vi "Version Utility - Top level.vi"() -> ()   [LabVIEW 2014]
uses:
  <vilib>/Utility/miscctls.llb/LVRowAndColumnTypeDef.ctl
  <vilib>/Utility/cursorutil.llb/Set Cursor (Icon Pict).vi
panel:
  in  "Open Button":bool
  in  "VI Paths and version information":i32(listbox)
  in  "Stop Button":bool
  out "Parent Path":path caption="selected path"
  out "Files Processed":i32
  out "file paths":path[](array[path])
  out "VI Versions":string[][](array[string])
  out "error out":errorcluster
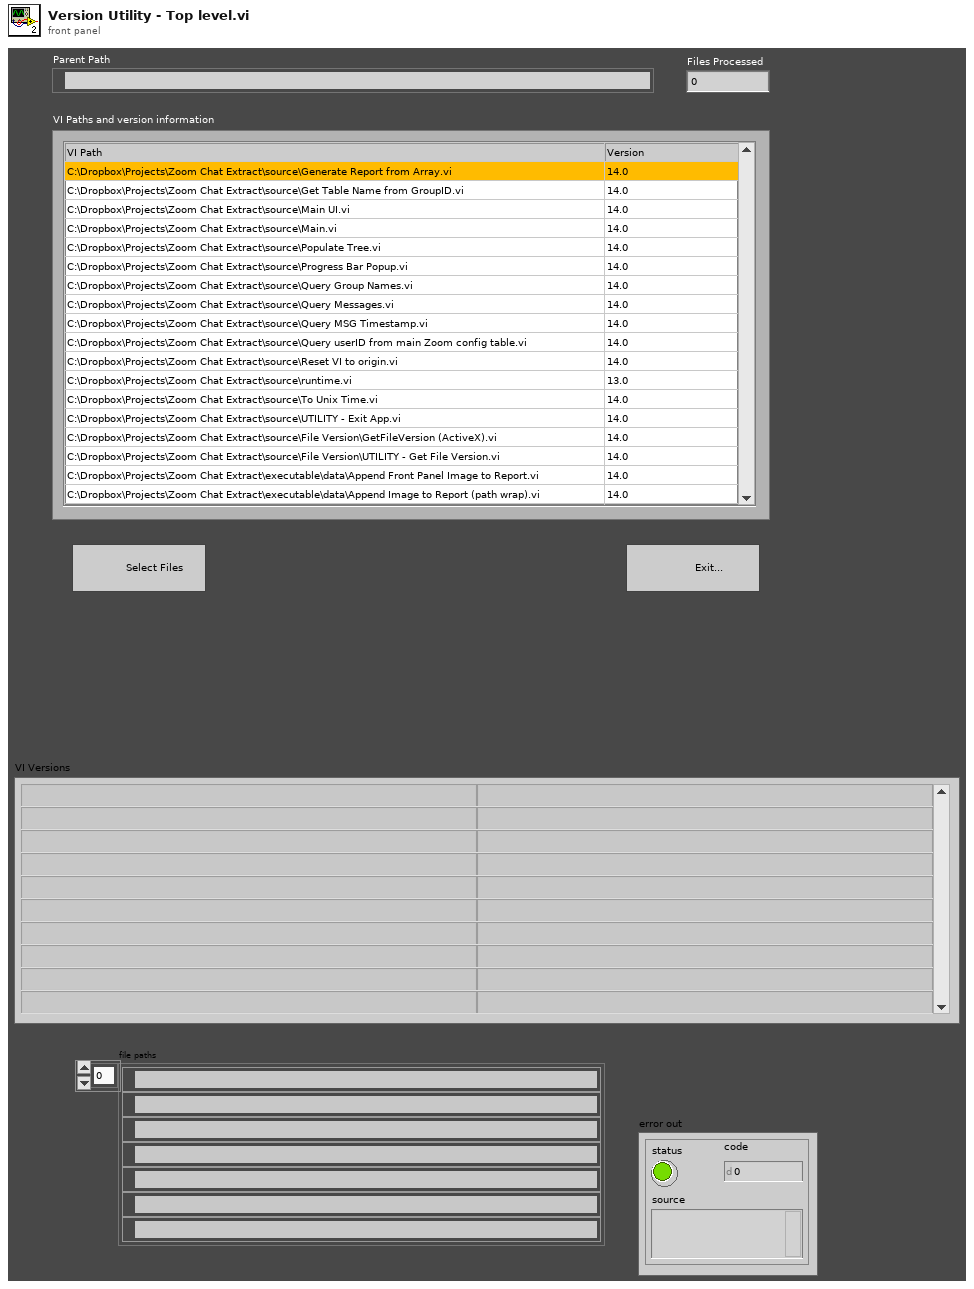
[diagram p1: front panel]
types:
  T1 = typedef "LVRowAndColumnTypeDef.ctl" = cluster{"Row":i32, "Column":i32}
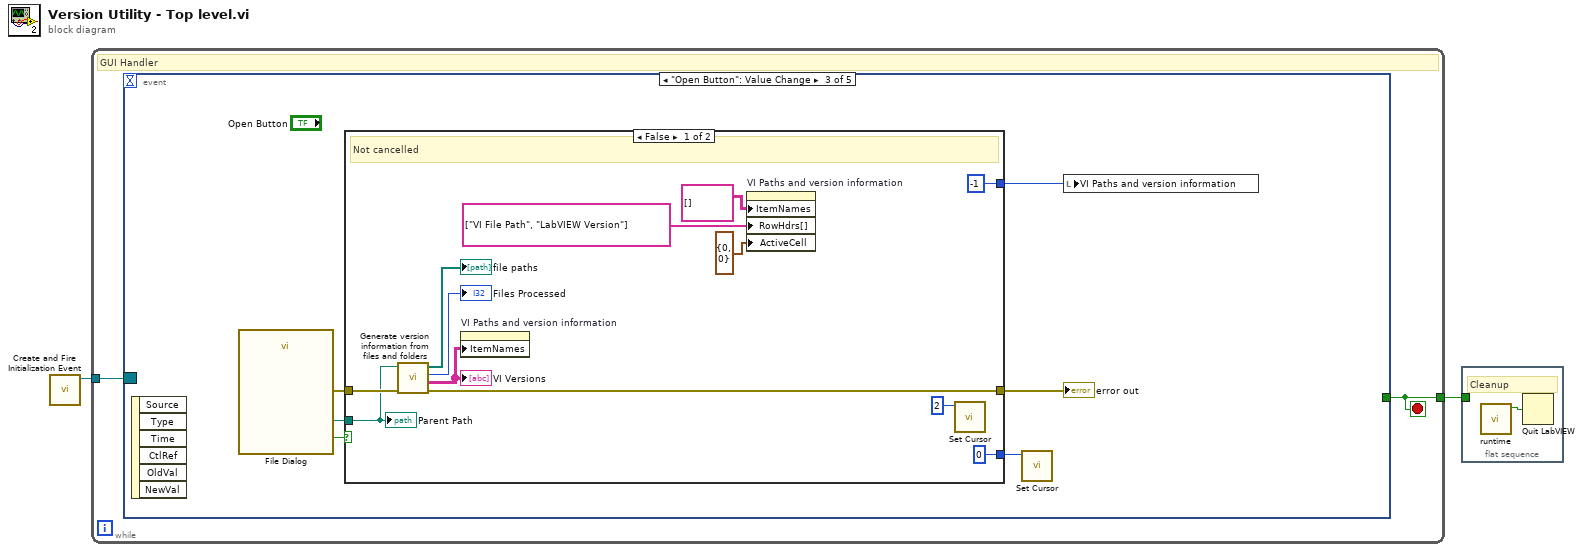
[diagram p0: block diagram]
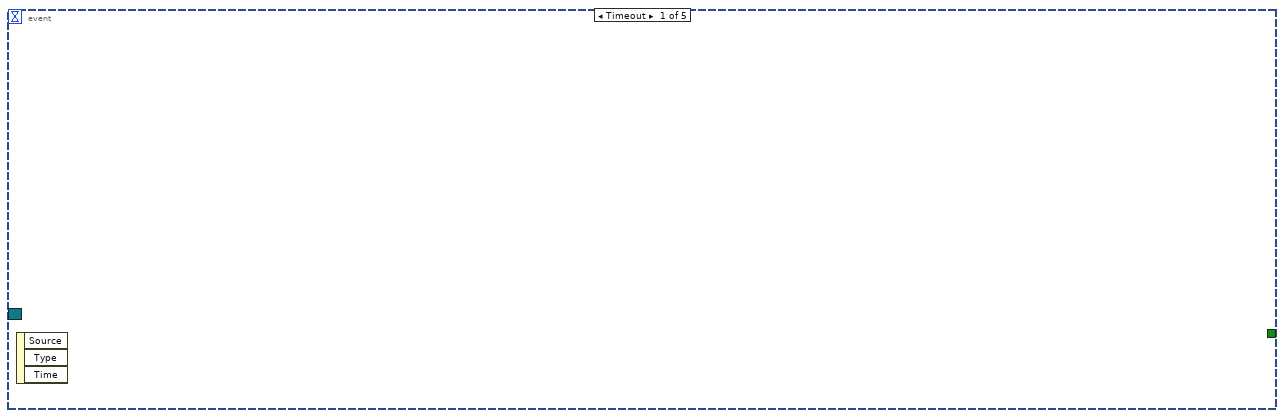
[diagram p2: hidden frame]
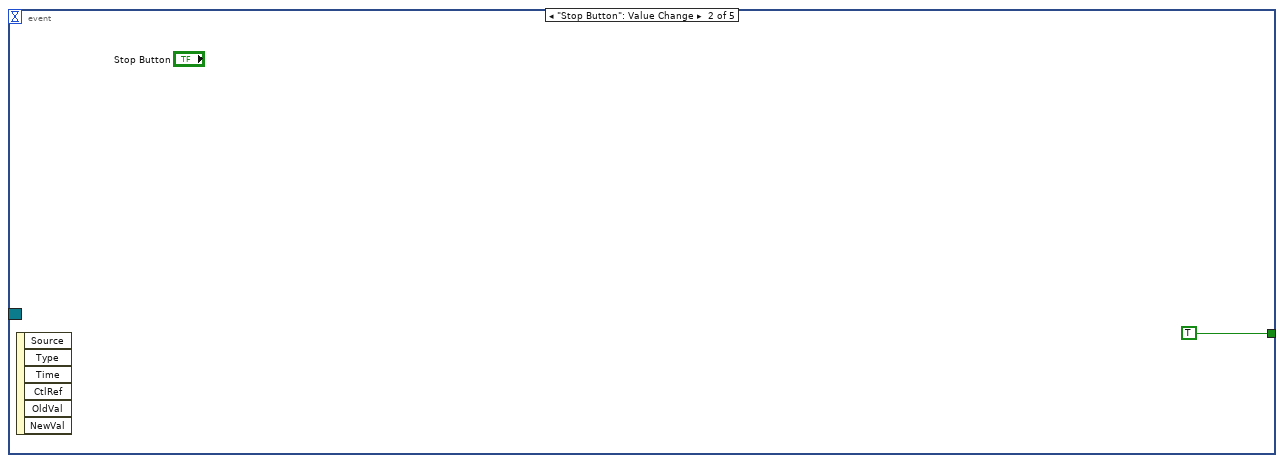
[diagram p3: hidden frame]
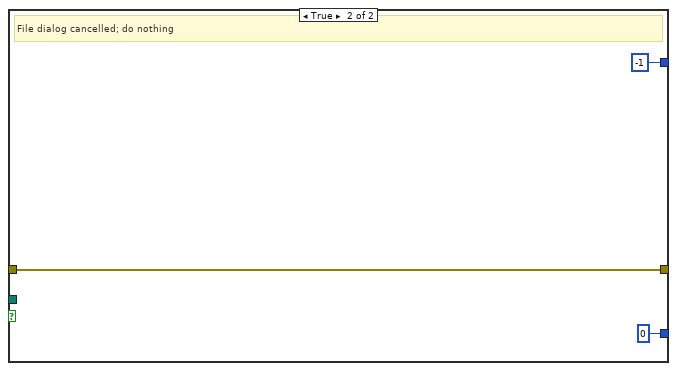
[diagram p4: hidden frame]
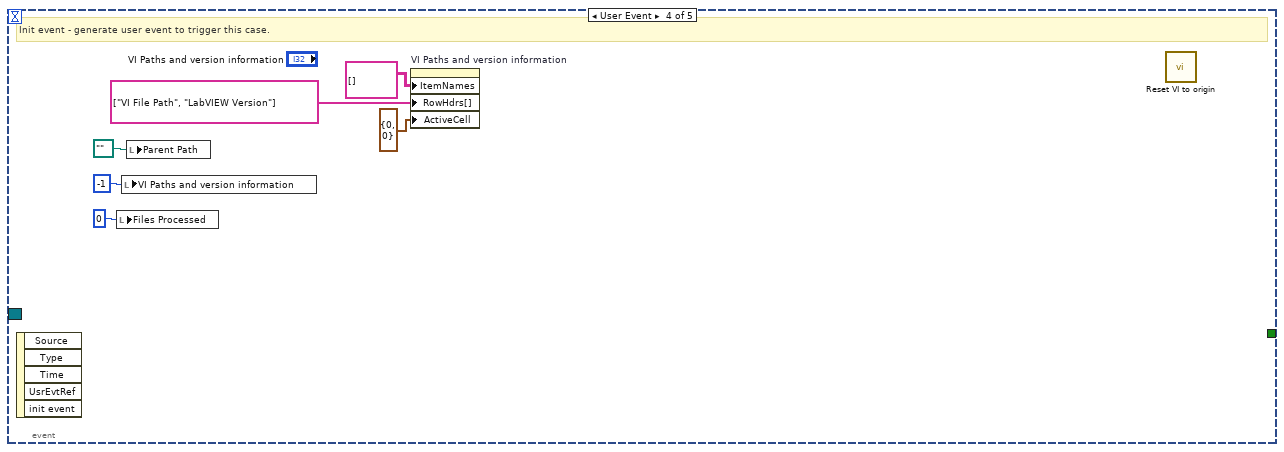
[diagram p5: hidden frame]
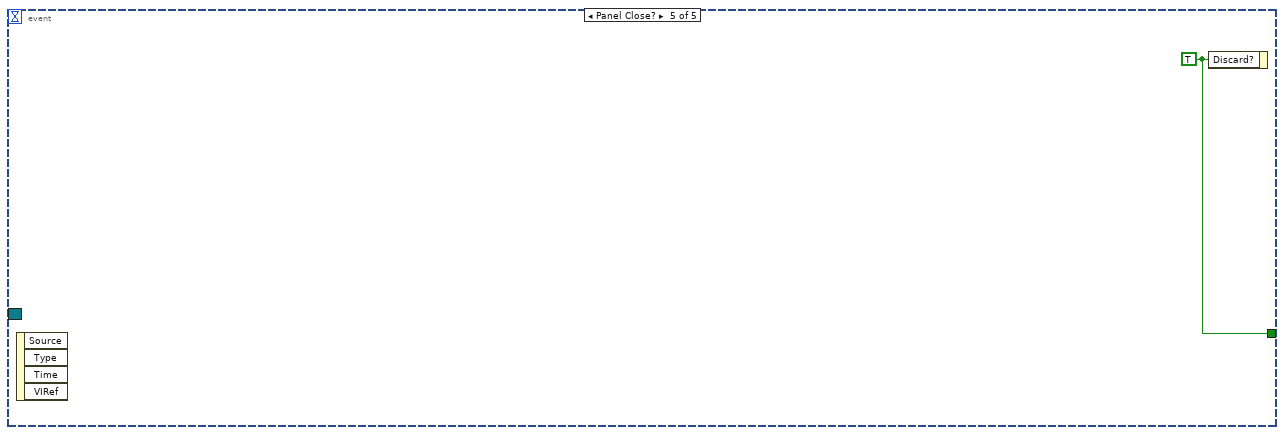
[diagram p6: hidden frame]
diagram:
  n1 = call "Create and Fire Initialization Event.vi"() -> ("Event Registration Refnum out"=w1:refnum<event-registration>)  [unwired: 11 in]
  n2 = while {
    tunnel: [w4] -> w2
    tunnel: w1 -> [w3]
    stop <- w4 stop-if-true
    # "GUI Handler"
    n3 = event shown="[2] \"Open Button\": Value Change" {
      selector: w3 -> [_ _ _ _ _]
      dyn-events: _ -> [_ _ _ _ _]
      timeout: _ -> [_ _ _ _ _]
      tunnel: [_ TRUE _ _ w33] -> w4
      event Timeout {
        n4 = event-data() -> ()  [unwired: 1 in, 3 out]
      }
      event "Stop Button": Value Change {
        n5 = event-data() -> ()  [unwired: 1 in, 6 out]
      }
      event "Open Button": Value Change {
        n6 = event-data() -> ()  [unwired: 1 in, 6 out]
        n7 = call "File Dialog"() -> ("selected path"=w8:path, "cancelled"=w9:bool, "error out"=w10:errorcluster)  [unwired: 12 in, 1 out]
        n8 = case shown="False" w9 {
          tunnel: [w23 w26] -> w11
          tunnel: w8 -> [w16 _]
          tunnel: w10 -> [w22 w26]
          tunnel: [u16 0 ("icon") u16 0 ("icon")] -> w7
          tunnel: [-1 ("Multicolumn Listbox") -1 ("Multicolumn Listbox")] -> w6
          frame False {
            # "Not cancelled"
            n9 = call "Generate version information from files and folders.vi"("error in (no error)"=w22, "selected path"=w16) -> ("error out"=w23:errorcluster, "Array"=w17:string[][], "Numeric Control"=→"Files Processed":i32, "file paths"=→"file paths":path[])  [unwired: 6 in]
            "VI Versions" <- w17
            n10 = property on="VI Paths and version information" class="MCListbox (strict)"("ItemNames"=w17) -> ()  [unwired: 2 in, 2 out]
            n11 = property on="VI Paths and version information" class="MCListbox (strict)"("ItemNames"=string[][] [] ("Item Names"), "RowHdrs[]"=string[] ["VI File Path", "LabVIEW Version"] ("Row Header Strings[]"), "ActiveCell"=T1 {"Row"=0, "Column"=0} ("Active Cell:Active Cell")) -> ()  [unwired: 2 in, 2 out]
            n12 = call-poly <vilib>:"Set Cursor.vi"("icon"=u16 2) -> ()  [unwired: 9 in, 2 out]
            "Parent Path" <- w16
          }
          frame True {
            # "File dialog cancelled; do nothing"
          }
        }
        "error out" <- w11
        n13 = call-poly <vilib>:"Set Cursor.vi"("icon"=w7) -> ()  [unwired: 9 in, 2 out]
        n14 = local write "VI Paths and version information"(w6) -> ()
      }
      event User Event {
        # "Init event - generate user event to trigger this case."
        n15 = event-data() -> ()  [unwired: 1 in, 5 out]
        n16 = local write "Files Processed"(0 ("Files Processed")) -> ()
        n17 = local write "VI Paths and version information"(-1 ("Multicolumn Listbox")) -> ()
        n18 = local write "Parent Path"(path "" ("Parent Path")) -> ()
        n19 = property on="VI Paths and version information" class="MCListbox (strict)"("ItemNames"=string[][] [] ("Item Names"), "RowHdrs[]"=string[] ["VI File Path", "LabVIEW Version"] ("Row Header Strings[]"), "ActiveCell"=T1 {"Row"=0, "Column"=0} ("Active Cell:Active Cell")) -> ()  [unwired: 2 in, 2 out]
        n20 = call "Reset VI to origin.vi"() -> ()  [unwired: 12 in]
      }
      event Panel Close? {
        w33 = TRUE ("Discard?")
        n21 = event-data() -> ()  [unwired: 1 in, 4 out]
        n22 = event-data("Discard?"=w33) -> ()  [unwired: 1 in, 1 out]
      }
    }
  }
  n23 = flat-sequence {
    tunnel: w2 -> [_]
    frame #0 {
      # "Cleanup"
      n24 = call "runtime.vi"() -> ("Runtime?"=w34:bool)  [unwired: 11 in]
      n25 = Quit LabVIEW(quit? (T)=w34) -> ()
    }
  }
